vi "__updateRoom.vi"(8 "room_device_type":T1, 9 "new_devices":string[](array[string]), 10 "roomGUID":string, 11 "Room-API In":refnum<class "Room-API.lvclass">) -> (0 "error out":errorcluster, 3 "Room-API out":refnum<class "Room-API.lvclass">)   [LabVIEW 2020, in "Room-API.lvclass"]
uses:
  Room-API.lvclass
  __room_device_type.ctl
  Room-API.lvclass/Room-API.ctl
  <userlib>/_OpenG.lib/array/array.llb/Remove Duplicates from 1D Array (String)__ogtk.vi
  <vilib>/ErrorRing/Error Ring.xnode
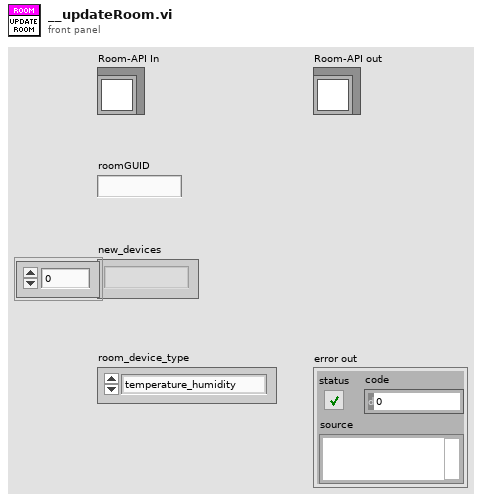
[diagram p1: front panel]
types:
  T1 = typedef "Room-API.lvclass/__room_device_type.ctl" = enum16{"temperature_humidity", "bond", "hue"}
  T2 = typedef "Room-API.lvclass/Single Room.ctl" = cluster{"name":string, "temperature_humidity":string[], "bond":string[], "hue":string[]}
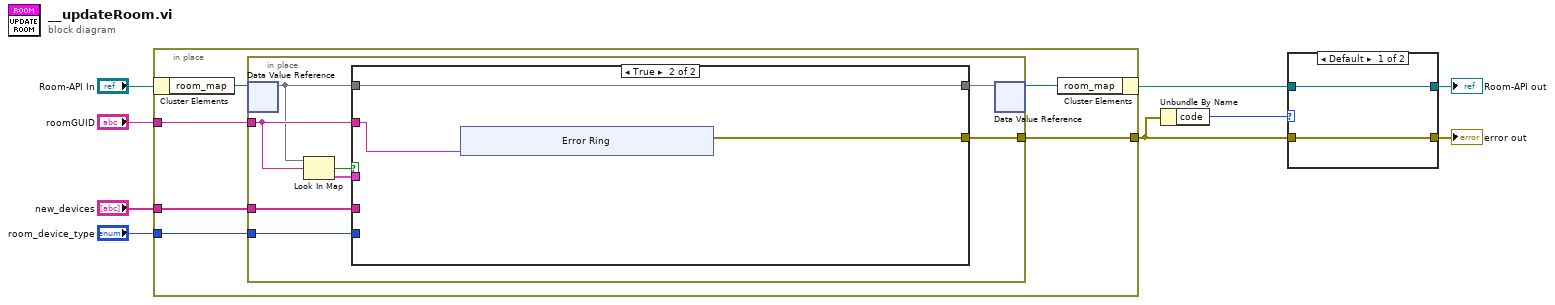
[diagram p0: block diagram]
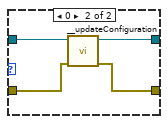
[diagram p2: hidden frame]
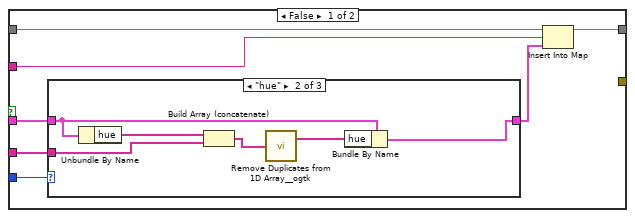
[diagram p3: hidden frame]
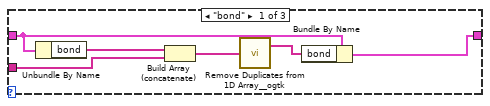
[diagram p4: hidden frame]
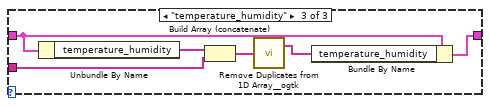
[diagram p5: hidden frame]
diagram:
  n1 = in-place {
    in-place-border: "new_devices" -> [w15]
    in-place-border: "roomGUID" -> [w14]
    in-place-border: "room_device_type" -> [w13]
    in-place-border: [w12] -> w2
    n2 = in-place-cluster #1("Room-API In") -> ("room_map"=w11:refnum<data-value>)
    n3 = in-place {
      in-place-border: w15 -> [w21]
      in-place-border: w14 -> [w20]
      in-place-border: w13 -> [w19]
      in-place-border: [w18] -> w12
      n4 = in-place-dvr #2(w11) -> (w17:map{string, T2})  [unwired: 1 out]
      n5 = Look In Map(map=w17, key=w20) -> (key not found?=w23:bool, value=w22:T2)  [unwired: 1 in]
      n6 = case shown="True" w23 {
        tunnel: w22 -> [w25 _]
        tunnel: w17 -> [w30 w51]
        tunnel: [w29 w51] -> w16
        tunnel: w21 -> [w26 _]
        tunnel: w20 -> [w28 w50]
        tunnel: w19 -> [w27 _]
        tunnel: [_ w49] -> w18
        frame False {
          n7 = case shown="\"hue\"" w27 {
            tunnel: w26 -> [w35 w41 w47]
            tunnel: w25 -> [w34 w40 w46]
            tunnel: [w33 w39 w44] -> w24
            frame "bond" {
              n8 = Unbundle By Name(w34) -> ("bond"=w36:string[])
              n9 = Build Array (concatenate)(w36, w35) -> (w32:string[])
              n10 = call-poly <userlib>:"Remove Duplicates from 1D Array__ogtk.vi"("Input Array"=w32) -> ("Output Array"=w31:string[])  [unwired: 1 out]
              n11 = Bundle By Name(cluster=w34, "bond"=w31) -> (w33:T2)
            }
            frame "hue" {
              n12 = Unbundle By Name(w40) -> ("hue"=w42:string[])
              n13 = Build Array (concatenate)(w42, w41) -> (w38:string[])
              n14 = call-poly <userlib>:"Remove Duplicates from 1D Array__ogtk.vi"("Input Array"=w38) -> ("Output Array"=w37:string[])  [unwired: 1 out]
              n15 = Bundle By Name(cluster=w40, "hue"=w37) -> (w39:T2)
            }
            frame "temperature_humidity" {
              n16 = Unbundle By Name(w46) -> ("temperature_humidity"=w48:string[])
              n17 = Build Array (concatenate)(w48, w47) -> (w45:string[])
              n18 = call-poly <userlib>:"Remove Duplicates from 1D Array__ogtk.vi"("Input Array"=w45) -> ("Output Array"=w43:string[])  [unwired: 1 out]
              n19 = Bundle By Name(cluster=w46, "temperature_humidity"=w43) -> (w44:T2)
            }
          }
          n20 = Insert Into Map(map in=w30, key=w28, value=w24) -> (map out=w29:map{string, T2})  [unwired: 2 out]
        }
        frame True {
          n21 = xnode "Error Ring"("parameter 0"=w50) -> ("error out"=w49:errorcluster)
        }
      }
      n22 = in-place-dvr #2(w16) -> (w10:refnum<data-value>)  [unwired: 1 out]
    }
    n23 = in-place-cluster #1("room_map"=w10) -> (w5:refnum<class "Room-API.lvclass">)
  }
  n24 = Unbundle By Name(w2) -> ("code"=w1:i32)
  n25 = case shown="Default" w1 {
    tunnel: w5 -> [w58 w62]
    tunnel: [w58 w61] -> w4
    tunnel: w2 -> [w57 w60]
    tunnel: [w57 w59] -> w3
    frame Default {
    }
    frame 0 {
      n26 = call "__updateConfiguration.vi"("error in (no error)"=w60, "Room-API in"=w62) -> ("error out"=w59:errorcluster, "Room-API out"=w61:refnum<class "Room-API.lvclass">)  [unwired: 8 in]
    }
  }
  "error out" <- w3
  "Room-API out" <- w4
